vi "CheckSet STOP(WithError).vi"(7 "stop value":bool, 9 "error in (no error)":errorcluster) -> (8 "Boolean":bool, 10 "error out":errorcluster)   [LabVIEW 2012, in "GlobalStop(dev).lvlib"]
uses:
  GlobalStop(dev).lvlib
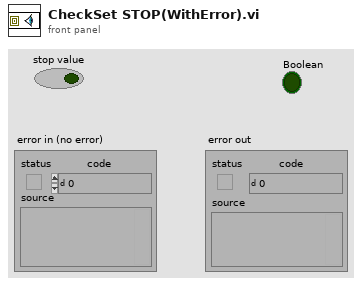
[diagram p1: front panel]
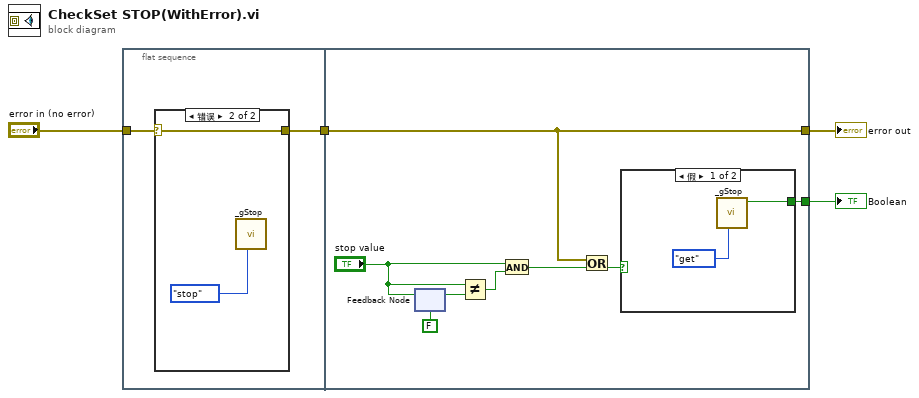
[diagram p0: block diagram]
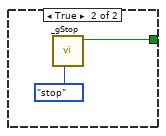
[diagram p3: hidden frame]
diagram:
  n1 = flat-sequence {
    tunnel: "error in (no error)" -> [w6]
    tunnel: [w5] -> w1
    tunnel: [w17] -> w4
    tunnel: [w10] -> w2
    tunnel: w1 -> [w10]
    frame #0 {
      n2 = case shown="错误" w6 {
        selector: w6 -> [w7 w8]
        tunnel: [w7 w8] -> w5
        frame No Error {
        }
        frame Error {
          n3 = call "_gStop.vi"("op"=enum16{"reset", "get", "stop"}."stop") -> ()  [unwired: 10 in, 1 out]
        }
      }
    }
    frame #1 {
      n4 = feedback #1(FALSE ("stop value")) -> (w15:bool)
      n5 = feedback-in #1("stop value") -> ()
      n6 = Not Equal?(x="stop value", y=w15) -> (x != y?=w14:bool)
      n7 = And(x="stop value", y=w14) -> (x .and. y?=w13:bool)
      n8 = Or(x=w10, y=w13) -> (x .or. y?=w11:bool)
      n9 = case shown="假" w11 {
        tunnel: [w19 w21] -> w17
        frame False {
          n10 = call "_gStop.vi"("op"=enum16{"reset", "get", "stop"}."get") -> ("Boolean"=w19:bool)  [unwired: 10 in]
        }
        frame True {
          n11 = call "_gStop.vi"("op"=enum16{"reset", "get", "stop"}."stop") -> ("Boolean"=w21:bool)  [unwired: 10 in]
        }
      }
    }
  }
  "error out" <- w2
  "Boolean" <- w4
